vi "Initialise All Aircraft Telemetry.vi"(8 "error IO":errorcluster) -> (0 "error out":errorcluster)   [LabVIEW 2014]
uses:
  Settings File/SubVI/Load Connection Type.vi
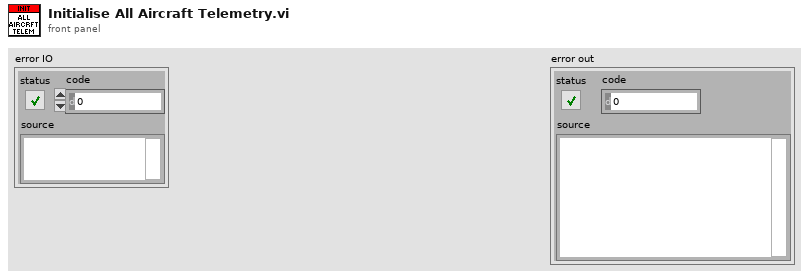
[diagram p1: front panel]
types:
  T1 = typedef "Telemetry Connection Type.ctl" = enum16{"Serial", "UDP", "TCP"}
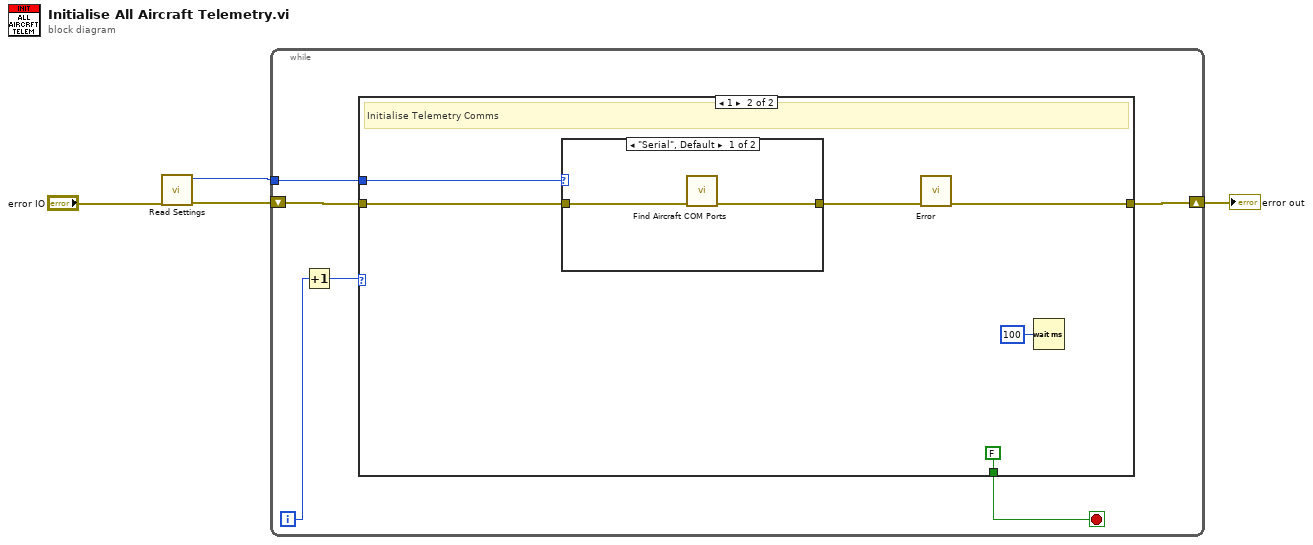
[diagram p0: block diagram]
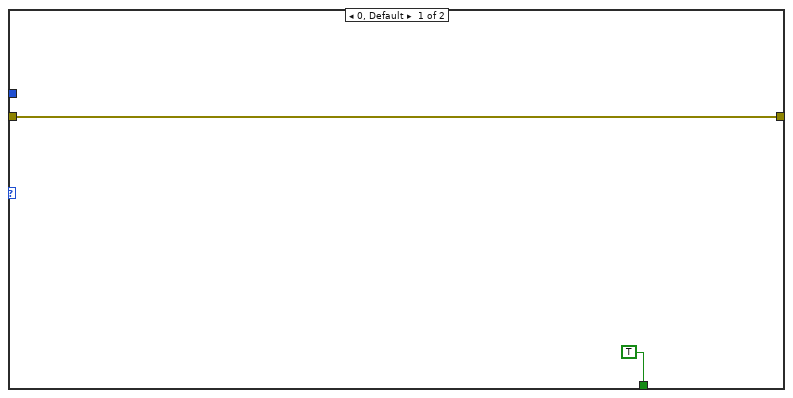
[diagram p2: hidden frame]
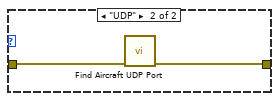
[diagram p3: hidden frame]
diagram:
  n1 = call-poly "Read Settings.vi"("Error In"="error IO") -> ("error out"=w2:errorcluster, "Connection Type"=w1:T1)  [unwired: 9 in]
  n2 = while {
    shift-right: [w9] -> w4
    shift-left: w2 -> [w8]
    tunnel: w1 -> [w5]
    i -> [w7]
    stop <- w10 stop-if-true
    n3 = Increment(x=w7) -> (x+1=w6:i32)
    n4 = case shown="1" w6 {
      tunnel: [TRUE FALSE] -> w10
      tunnel: [w11 w16] -> w9
      tunnel: w8 -> [w11 w17]
      tunnel: w5 -> [_ w13]
      frame 0, Default {
      }
      frame 1 {
        # "Initialise Telemetry Comms"
        n5 = case shown="\"Serial\", Default" w13 {
          tunnel: w17 -> [w20 w22]
          tunnel: [w19 w21] -> w15
          frame "Serial", Default {
            n6 = call "Find Aircraft COM Ports.vi"("Error In"=w20) -> ("Error Out"=w19:errorcluster)  [unwired: 9 in, 1 out]
          }
          frame "UDP" {
            n7 = call "Find Aircraft UDP Port.vi"("Error In"=w22) -> ("Error Out"=w21:errorcluster)  [unwired: 9 in, 1 out]
          }
        }
        n8 = call "Error.vi"("Error In"=w15) -> ("Error Out"=w16:errorcluster)  [unwired: 10 in]
        n9 = Wait (ms)(milliseconds to wait=u32 100) -> ()  [unwired: 1 out]
      }
    }
  }
  "error out" <- w4
